vi "수업.vi"() -> ()   [LabVIEW 2014]
panel:
  out "배열":dbl[](array[numeric])
  out "동작":bool
  out "숫자형":i32
  in  "정지":bool
  in  "다이얼":dbl(knob) scale=0.0..1000.0
  out "웨이브폼 차트":dbl(graph)
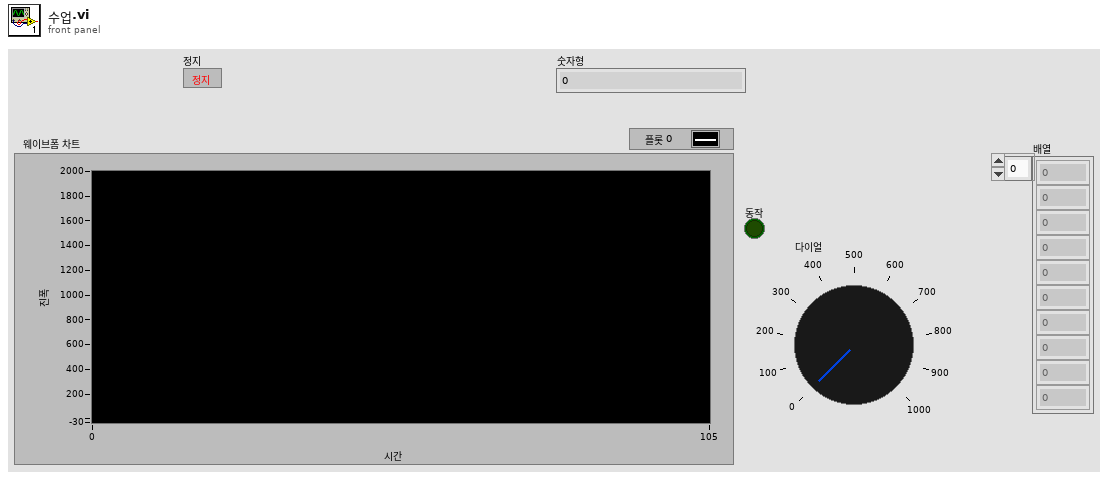
[diagram p1: front panel]
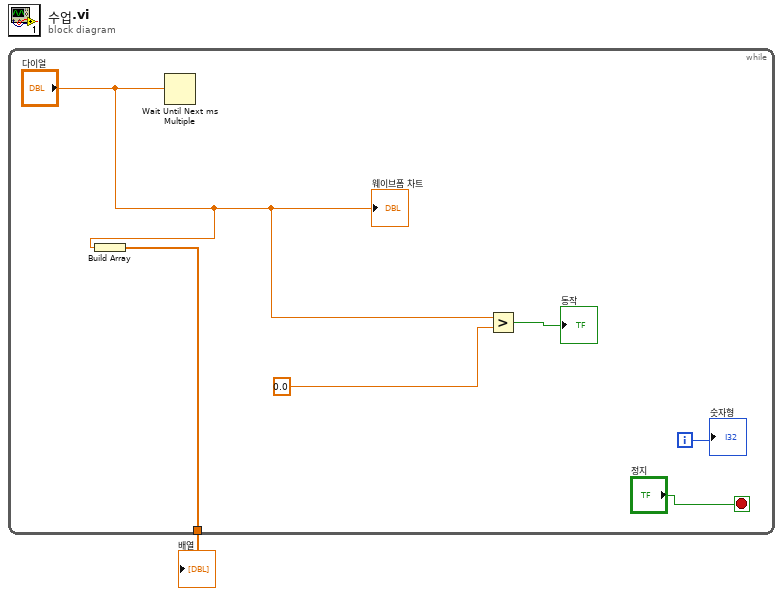
[diagram p0: block diagram]
diagram:
  n1 = while {
    tunnel: [w3] -> w1
    i -> [w6]
    stop <- "정지" stop-if-true
    n2 = Build Array("다이얼") -> (w3:dbl[])
    n3 = Wait Until Next ms Multiple(millisecond multiple="다이얼") -> ()  [unwired: 1 out]
    n4 = Greater?(x="다이얼", y=0.0) -> (0:→"동작":bool)
    "웨이브폼 차트" <- "다이얼"
    "숫자형" <- w6
  }
  "배열" <- w1
